vi "Close DSF Configuration Data.vi"(6 "version (no change)":T1, 8 "error in (no error)":errorcluster, 10 "write file if changed (T)":bool=TRUE, 11 "dsf refnum":T2) -> (0 "error out":errorcluster, 3 "file path":path)   [LabVIEW 2017, in "DSF Core.lvlib"]
doc: "Writes data to the platform-independent configuration file identified by <B>dsf refnum</B> and then closes the reference to that file."
uses:
  DSF Core.lvlib
  Controls/DSF Config Data RefNum.ctl
  Controls/DSF Version Info.ctl
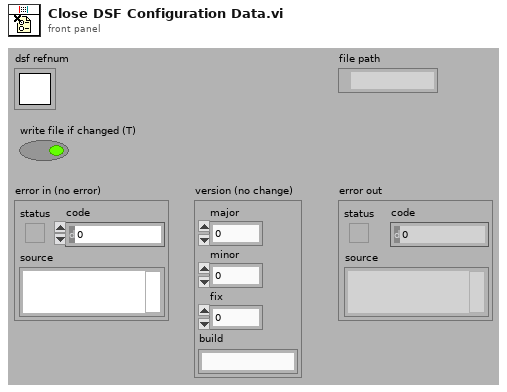
[diagram p1: front panel]
types:
  T1 = typedef "DSF Core.lvlib/DSF Version Info.ctl" = cluster{"major":u32, "minor":u32, "fix":u32, "build":string}
  T2 = typedef "DSF Core.lvlib/DSF Config Data RefNum.ctl" = refnum<k1>
  T3 = typedef "DSF Core.lvlib/DSF Configuration Reference.ctl" = refnum<data-value>
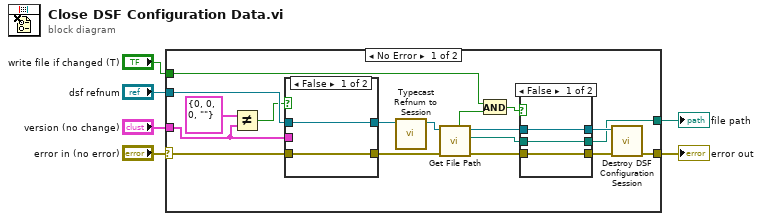
[diagram p0: block diagram]
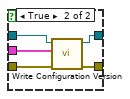
[diagram p2: hidden frame]
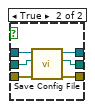
[diagram p3: hidden frame]
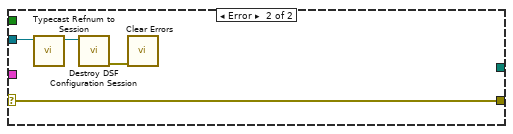
[diagram p4: hidden frame]
diagram:
  n1 = case shown="No Error" "error in (no error)" {
    selector: "error in (no error)" -> [w21 w44]
    tunnel: "dsf refnum" -> [w11 w43]
    tunnel: "write file if changed (T)" -> [w23 _]
    tunnel: [w18 w44] -> w4
    tunnel: [w13 _] -> w3
    tunnel: "version (no change)" -> [w7 _]
    frame No Error {
      n2 = Not Equal?(x=T1 {"major"=0, "minor"=0, "fix"=0, "build"=""} ("version"), y=w7) -> (x != y?=w8:bool)
      n3 = case shown="False" w8 {
        tunnel: w21 -> [w25 w31]
        tunnel: [w25 w30] -> w12
        tunnel: w11 -> [w26 w29]
        tunnel: [w26 w28] -> w10
        tunnel: w7 -> [_ w27]
        frame False {
        }
        frame True {
          n4 = call "Write Configuration Version.vi"("error in (no error)"=w31, "Configuration Version"=w27, "dsf refnum"=w29) -> ("error out"=w30:errorcluster, "dsf refnum out"=w28:T2)  [unwired: 7 in]
        }
      }
      n5 = call "Typecast Refnum to Session.vi"("dsf refnum in"=w10) -> ("DSF Configuration Session out"=w17:T3)  [unwired: 10 in]
      n6 = call "Get File Path.vi"("error in (no error)"=w12, "DSF Configuration Reference in"=w17) -> ("error out"=w15:errorcluster, "file path"=w14:path, "DSF Configuration Reference out"=w22:T3, "need update"=w16:bool)  [unwired: 1 in, 5 out]
      n7 = And(x=w23, y=w16) -> (x .and. y?=w24:bool)
      n8 = case shown="False" w24 {
        tunnel: w15 -> [w34 w40]
        tunnel: w22 -> [w33 w35]
        tunnel: [w34 w39] -> w19
        tunnel: [w33 w38] -> w20
        tunnel: w14 -> [w32 w37]
        tunnel: [w32 w36] -> w13
        frame False {
        }
        frame True {
          n9 = call "Save Config File.vi"("error in (no error)"=w40, "file path"=w37, "DSF Configuration Reference in"=w35) -> ("error out"=w39:errorcluster, "file path out"=w36:path, "DSF Configuration Reference out"=w38:T3)  [unwired: 6 out]
        }
      }
      n10 = call "Destroy DSF Configuration Session.vi"("error in (no error)"=w19, "DSF Configuration Session in"=w20) -> ("error out"=w18:errorcluster)  [unwired: 9 in]
    }
    frame Error {
      n11 = call "Typecast Refnum to Session.vi"("dsf refnum in"=w43) -> ("DSF Configuration Session out"=w42:T3)  [unwired: 10 in]
      n12 = call "Destroy DSF Configuration Session.vi"("DSF Configuration Session in"=w42) -> ("error out"=w41:errorcluster)  [unwired: 10 in]
      n13 = call <vilib>:"Clear Errors.vi"("error in (no error)"=w41) -> ()  [unwired: 5 in, 2 out]
    }
  }
  "error out" <- w4
  "file path" <- w3
